vi "set invoke node.vi"(8 "error in":errorcluster, 9 "object_id":string, 11 "method_name":string) -> (0 "error out":errorcluster)   [LabVIEW 2020]
doc: "Selects which method an already-placed Invoke Node calls, since add_object_to_vi cannot pick a method by itself.\n \nFirst wire the target class's reference (VI, Application, Project, Control, etc.) into the Invoke Node's reference input, then call get_available_methods on that same object_id to list the class's methods. \n\nSet method_name to the \"Unique ID string\" field from that list (e.g. \"7d5\" for the Application class's Mass Compile method) — this is the reliable exact match. \n\nThe \"Data name\"/display text (e.g. \"Mass Compile\") is not the same string internally and will error (code 1077).\n\nAfter this call succeeds, use get_object_terminals on the same object_id to discover the method's parameter and return terminals, then wire them with connect_objects or create controls with create_control as usual."
uses:
  G-AI Core/G-AI Core.lvlib
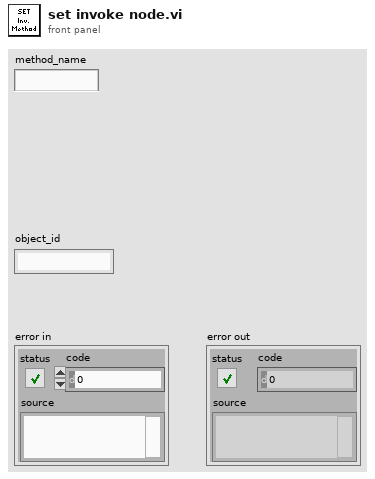
[diagram p1: front panel]
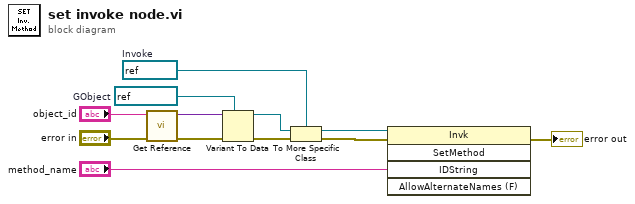
[diagram p0: block diagram]
diagram:
  w6 = refnum<vi> refnum  # Invoke
  w7 = refnum<vi> refnum  # GObject
  n1 = call "Get Reference.vi"("error in"="error in", "id"="object_id") -> ("error out"=w10:errorcluster, "reference"=w9:variant)  [unwired: 8 in]
  n2 = Variant To Data(error in=w10, type=w7, Variant=w9) -> (data=w5:refnum<vi>, error out=w8:errorcluster)
  n3 = To More Specific Class(target class=w6, reference=w5, error in=w8) -> (specific class reference=w3:refnum<vi>, error out=w4:errorcluster)
  n4 = invoke class="Invk" method="SetMethod"(reference=w3, error in=w4, "IDString"="method_name") -> (error out=→"error out":errorcluster)  [unwired: 2 in, 4 out]
